vi "run_folder.vi"() -> ()   [LabVIEW 2014]
panel:
  in  "Folder Path":path
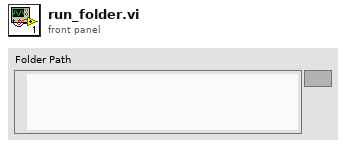
[diagram p1: front panel]
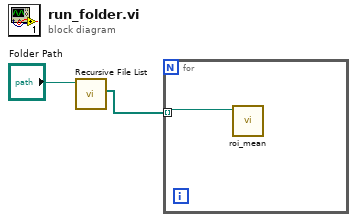
[diagram p0: block diagram]
diagram:
  n1 = call <vilib>:"Recursive File List.vi"("Folder Path"="Folder Path") -> ("All Files in Dir"=w1:path[])  [unwired: 6 in, 4 out]
  n2 = for {
    tunnel: w1 -> [w3] mode=indexing
    n3 = call "roi_mean.vi"("file (use dialog)"=w3) -> ()  [unwired: 11 in]
  }
